vi "Construct ModelTimesNObservations.vi"(10 "Stop After N Observations":i32) -> (1 "Elaped Seconds":refnum<notifier>, 3 "ModelCountsObservations Out":refnum<class "ModelTimesNObservations.lvclass">)   [LabVIEW 2017, in "BenchmarkObservationRate.lvlib" / "ModelTimesNObservations.lvclass"]
uses:
  ModelTimesNObservations.lvclass
  ModelTimesNObservations.lvclass/ModelTimesNObservations.ctl
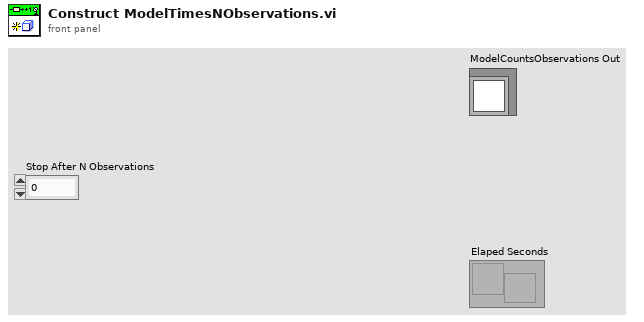
[diagram p1: front panel]
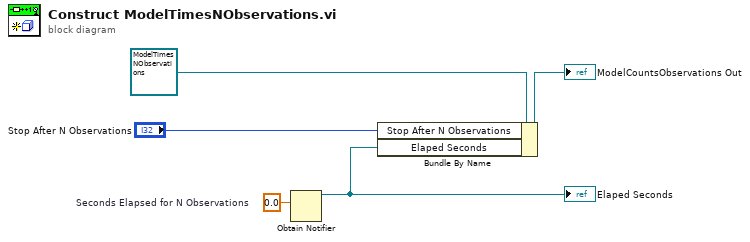
[diagram p0: block diagram]
diagram:
  w3 = 0.0  # Seconds Elapsed for N Observations
  n1 = Obtain Notifier(notification data type=w3) -> (notifier out=w2:refnum<notifier>)  [unwired: 3 in, 2 out]
  "Elaped Seconds" <- w2
  n2 = Bundle By Name(cluster=refnum<class "ModelTimesNObservations.lvclass"> refnum ("RootModelNotifiesWhenStopped in"), "Stop After N Observations"="Stop After N Observations", "Elaped Seconds"=w2) -> (→"ModelCountsObservations Out":refnum<class "ModelTimesNObservations.lvclass">)
